vi "Simple_DAQ_AnalogIO.i attribute.vi"(0 "VI Refnum":refnum<vi>, 2 "CLASS.i attribute":T1, 3 "Action":T2(ring), 5 "error in (no error)":errorcluster) -> (14 "VI Refnum out":refnum<vi>, 16 "CLASS.i attribute out":T1, 19 "error out":errorcluster)   [LabVIEW 2014, in "Simple_DAQ_AnalogIO.lvlib"]
doc: "This is a so-called functional global variable. It manages the access to a global variable in a thread-safe way. \n\nHere the attribute data of all instances of THIS class are stored. This is done for performance reasons.\n\nLicense Agreement for this software:\n\nCopyright (C)\nGesellschaft für Schwerionenforschung, GSI\nPlanckstr. 1\n64291 Darmstadt\nGermany\n\nContact: D.Beck@gsi.de \n\nThis program is free software; you can redistribute it and/or modify it under the terms of the GNU General Public License as published by the Free Software Foundation; either version 2 of the license, or (at your option) any later version.\n\nThis program is distributed in the hope that it will be useful, but WITHOUT ANY WARRANTY; without even the implied warranty of MERCHANTABILITY or FITNESS FOR A PARTICULAR PURPOSE. See the GNU General License for more details (http://www.gnu.org).\n\nGesellschaft für Schwerionenforschung, GSI\nPlanckstr. 1, 64291 Darmstadt, Germany\nFor all questions and ideas contact: M.Richter@gsi.de, H.Brand@gsi.de or D.Beck@gsi.de.\nLast update: 17-JUN-2004"
uses:
  Simple_DAQ_AnalogIO.lvlib
  Simple_DAQ_AnalogIO.i attribute.ctl
  CS_Core/CSSystem/CoreDefs/CoreDefs.error_type.ctl
  CS_Core/CSSystem/CoreLib/CoreLib.lvlib
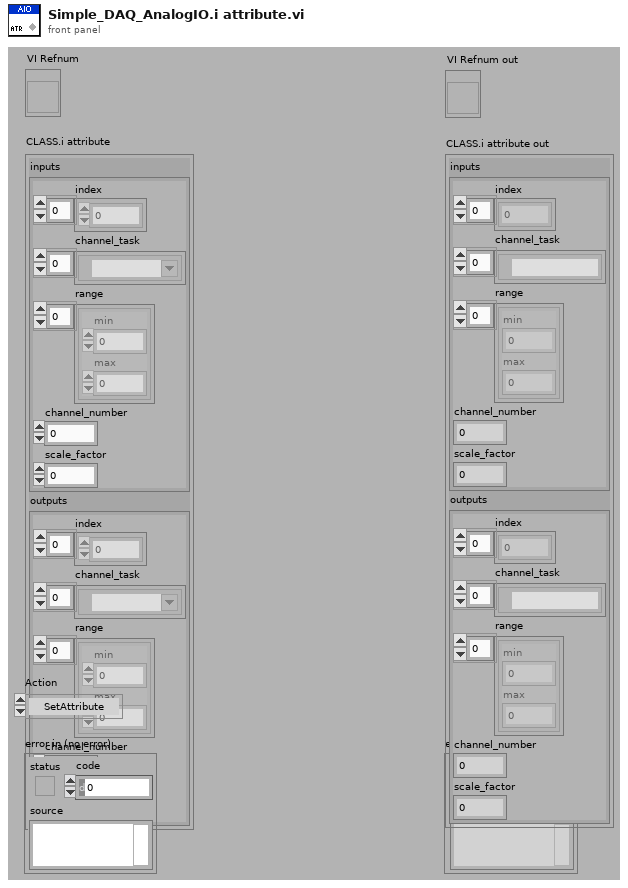
[diagram p1: front panel]
types:
  T1 = typedef "Simple_DAQ_AnalogIO.lvlib/Simple_DAQ_AnalogIO.i attribute.ctl" = cluster{"inputs":cluster{"index":i32[], "channel_task":refnum<k21>[], "range":cluster{"min":dbl, "max":dbl}[], "channel_number":i32, "scale_factor":dbl}, "outputs":cluster{"index":i32[], "channel_task":refnum<k21>[], "range":cluster{"min":dbl, "max":dbl}[], "channel_number":i32, "scale_factor":dbl}}
  T2 = enum16{"SetAttribute", "GetAttribute", "CreateAttribute", "DestroyAttribute", "DestroyAllAtributes"}
  T3 = typedef "CoreDefs.error_type.ctl" = enum16{"no error", "can't load process", "can't unload process", "process does not exist", "can't install process", "can't remove process", "unknown function", "time out", "can't execute function", "duplicate queue name", "super not found", "caller queue invalid", "can't ping process", "unknown error", "VISA Error", "VISA timeout", "GPIB timeout", "GPIB error", "communication error", "data type mismatch", "can't read data from OPC server", "can't write data to OPC server", "OET error", "function not implemented", "process already exists", "invalid Shared Variable name", "error writing Shared Variable", "error reading Shared Variable", "invalid client name", "corrupt database", "unknown class", "call not authorized", "parameter out of range", "OET timeout: can't get data to modify", "invalid queue name", "requested operation incompatible with current state", "event undefined", "event disabled", "state undefined", "caller is not a friend", "EventBuilder: bad eventID", "EventBuilder: no DAQ devices", "a thread must not stop itself", "UNUSED ELEMENT4", "DiscArchiver: eventData incomplete", "DiscArchiver: eventData does not belong to run", "DiscArchiver: can't open file", "DiscArchiver: can't write to file", "DiscArchiver: available disc space low", "can't acquire semaphore", "error reading data from database", "notifier object is not existing", "can't register process", "can't unregister process", "illegal event type", "object disabled", "object already exists", "can't change state", "Instrument not found", "no connection to remote node", "invalid reference", "N/A", "UNUSED ELEMENT 1", "element not found", "illegal TCP/IP connection detected", "object does not exist", "invalid access ID", "unknown CS system", "invalid privilige", "unsupported data type", "unsupported server type", "IO server already exists", "Shared Variable already exists"}
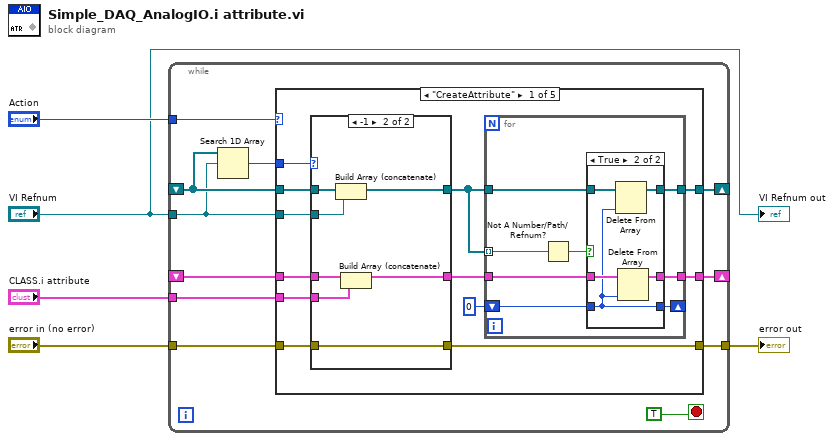
[diagram p0: block diagram]
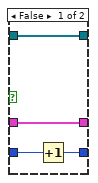
[diagram p2: hidden frame]
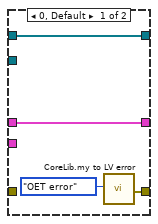
[diagram p3: hidden frame]
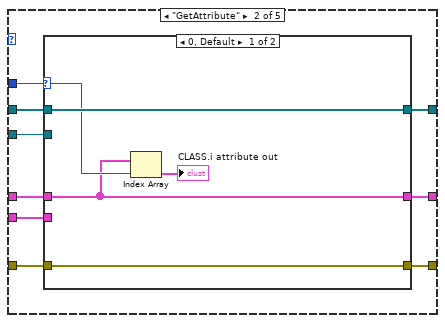
[diagram p4: hidden frame]
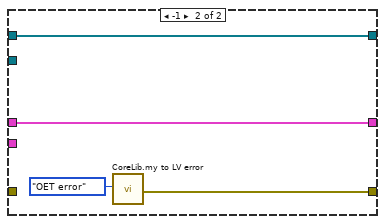
[diagram p5: hidden frame]
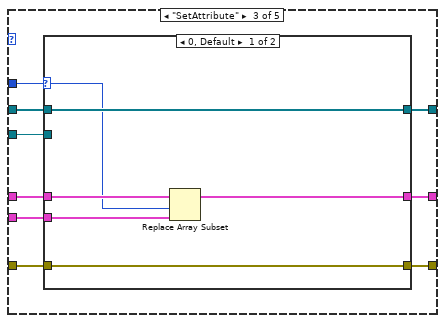
[diagram p6: hidden frame]
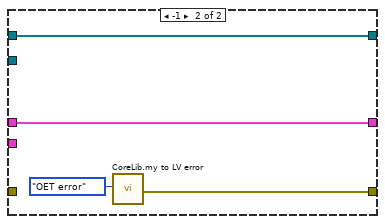
[diagram p7: hidden frame]
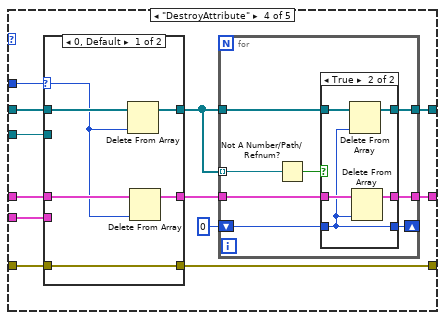
[diagram p8: hidden frame]
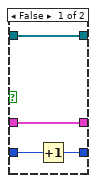
[diagram p9: hidden frame]
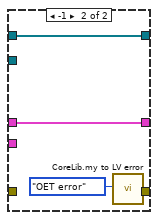
[diagram p10: hidden frame]
diagram:
  n1 = while {
    shift-right: [w10] -> _
    shift-left: _ -> [w11]
    tunnel: "Action" -> [w15]
    shift-right: [w12] -> _
    shift-left: _ -> [w8]
    tunnel: "VI Refnum" -> [w7]
    tunnel: "error in (no error)" -> [w14]
    tunnel: [w13] -> w3
    tunnel: "CLASS.i attribute" -> [w9]
    stop <- TRUE stop-if-true
    n2 = Search 1D Array(1D array=w8, element=w7) -> (index of element=w6:i32)  [unwired: 1 in]
    n3 = case shown="\"CreateAttribute\"" w15 {
      tunnel: w8 -> [w26 w63 w81 w103 _]
      tunnel: w7 -> [w25 w61 w79 w102 _]
      tunnel: w14 -> [w28 w65 w83 w105 w133]
      tunnel: [w27 w64 w82 w104 w133] -> w13
      tunnel: [w20 w62 w80 w97 _] -> w12
      tunnel: w11 -> [w24 w60 w78 w101 _]
      tunnel: [w19 w59 w77 w95 _] -> w10
      tunnel: w9 -> [w23 w58 w76 w100 _]
      tunnel: w6 -> [w22 w57 w75 w99 _]
      frame "CreateAttribute" {
        n4 = case shown="-1" w22 {
          tunnel: w28 -> [_ w56]
          tunnel: [w48 w56] -> w27
          tunnel: w26 -> [w47 w55]
          tunnel: [w47 w54] -> w18
          tunnel: w25 -> [_ w53]
          tunnel: w24 -> [w46 w52]
          tunnel: [w46 w51] -> w17
          tunnel: w23 -> [_ w50]
          frame 0, Default {
            n5 = call "CoreLib.my to LV error.vi"("ErrorTypes"=CoreDefs.error_type."OET error") -> ("myErrorCluster"=w48:errorcluster)  [unwired: 17 in, 1 out]
          }
          frame -1 {
            n6 = Build Array (concatenate)(w55, w53) -> (w54:refnum<vi>[])
            n7 = Build Array (concatenate)(w52, w50) -> (w51:T1[])
          }
        }
        n8 = for {
          tunnel: w18 -> [w33]
          tunnel: [w32] -> w20
          tunnel: [w36] -> w19
          tunnel: w17 -> [w35]
          tunnel: w18 -> [w31] mode=indexing
          shift-right: [w30] -> _
          shift-left: 0 -> [w29]
          n9 = Not A Number/Path/Refnum?(number/path/refnum=w31) -> (NaN/Path/Refnum?=w34:bool)
          n10 = case shown="True" w34 {
            tunnel: [w40 w45] -> w36
            tunnel: w35 -> [w40 w44]
            tunnel: [w39 w42] -> w32
            tunnel: w33 -> [w39 w43]
            tunnel: w29 -> [w38 w41]
            tunnel: [w37 w41] -> w30
            frame False {
              n11 = Increment(x=w38) -> (x+1=w37:i32)
            }
            frame True {
              n12 = Delete From Array(array=w43, index=w41) -> (array with subset deleted=w42:refnum<vi>[])  [unwired: 1 in, 1 out]
              n13 = Delete From Array(array=w44, index=w41) -> (array with subset deleted=w45:T1[])  [unwired: 1 in, 1 out]
            }
          }
        }
      }
      frame "GetAttribute" {
        n14 = case shown="0, Default" w57 {
          selector: w57 -> [w68 _]
          tunnel: w65 -> [w70 _]
          tunnel: [w70 w73] -> w64
          tunnel: w63 -> [w69 w72]
          tunnel: [w69 w72] -> w62
          tunnel: w61 -> [_ _]
          tunnel: w60 -> [w67 w71]
          tunnel: [w67 w71] -> w59
          tunnel: w58 -> [_ _]
          frame 0, Default {
            n15 = Index Array(array=w67, index=w68) -> (element=→"CLASS.i attribute out":T1)
          }
          frame -1 {
            n16 = call "CoreLib.my to LV error.vi"("ErrorTypes"=CoreDefs.error_type."OET error") -> ("myErrorCluster"=w73:errorcluster)  [unwired: 17 in, 1 out]
          }
        }
      }
      frame "SetAttribute" {
        n17 = case shown="0, Default" w75 {
          selector: w75 -> [w85 _]
          tunnel: w83 -> [w89 _]
          tunnel: [w89 w92] -> w82
          tunnel: w81 -> [w88 w91]
          tunnel: [w88 w91] -> w80
          tunnel: w79 -> [_ _]
          tunnel: w78 -> [w87 w90]
          tunnel: [w86 w90] -> w77
          tunnel: w76 -> [w84 _]
          frame 0, Default {
            n18 = Replace Array Subset(array=w87, new element=w84, index=w85) -> (w86:T1[])
          }
          frame -1 {
            n19 = call "CoreLib.my to LV error.vi"("ErrorTypes"=CoreDefs.error_type."OET error") -> ("myErrorCluster"=w92:errorcluster)  [unwired: 17 in, 1 out]
          }
        }
      }
      frame "DestroyAttribute" {
        n20 = case shown="0, Default" w99 {
          selector: w99 -> [w124 _]
          tunnel: w105 -> [w128 _]
          tunnel: [w128 w131] -> w104
          tunnel: w103 -> [w127 w130]
          tunnel: [w126 w130] -> w96
          tunnel: w102 -> [_ _]
          tunnel: w101 -> [w125 w129]
          tunnel: [w123 w129] -> w94
          tunnel: w100 -> [_ _]
          frame 0, Default {
            n21 = Delete From Array(array=w127, index=w124) -> (array with subset deleted=w126:refnum<vi>[])  [unwired: 1 in, 1 out]
            n22 = Delete From Array(array=w125, index=w124) -> (array with subset deleted=w123:T1[])  [unwired: 1 in, 1 out]
          }
          frame -1 {
            n23 = call "CoreLib.my to LV error.vi"("ErrorTypes"=CoreDefs.error_type."OET error") -> ("myErrorCluster"=w131:errorcluster)  [unwired: 17 in, 1 out]
          }
        }
        n24 = for {
          tunnel: w96 -> [w110]
          tunnel: [w109] -> w97
          tunnel: [w113] -> w95
          tunnel: w94 -> [w112]
          tunnel: w96 -> [w108] mode=indexing
          shift-right: [w107] -> _
          shift-left: 0 -> [w106]
          n25 = Not A Number/Path/Refnum?(number/path/refnum=w108) -> (NaN/Path/Refnum?=w111:bool)
          n26 = case shown="True" w111 {
            tunnel: [w117 w122] -> w113
            tunnel: w112 -> [w117 w121]
            tunnel: [w116 w119] -> w109
            tunnel: w110 -> [w116 w120]
            tunnel: w106 -> [w115 w118]
            tunnel: [w114 w118] -> w107
            frame False {
              n27 = Increment(x=w115) -> (x+1=w114:i32)
            }
            frame True {
              n28 = Delete From Array(array=w120, index=w118) -> (array with subset deleted=w119:refnum<vi>[])  [unwired: 1 in, 1 out]
              n29 = Delete From Array(array=w121, index=w118) -> (array with subset deleted=w122:T1[])  [unwired: 1 in, 1 out]
            }
          }
        }
      }
      frame "DestroyAllAtributes" {
      }
    }
  }
  "error out" <- w3
  "VI Refnum out" <- "VI Refnum"
